vi "HAMEG_HMP2020.vi"() -> ()   [LabVIEW 2009, in "run.lvlib"]
uses:
  run.lvlib
panel:
  in  "Time":dbl[](array[numeric])
  in  "Voltage":dbl[](array[numeric])=[2.0, 2.0] format="%.3f"
  in  "Current":dbl[](array[numeric]) format="%.3f"
  in  "Channel (Channel 1)":i32(ring)=1 items=["Channel 1"=1, "Channel 2"=2, "Channel 3"=3, "Channel 4"=4]
  in  "VISA resource name":refnum<visa-resource-name>="GPIB::20::INSTR"
  in  "stop":bool
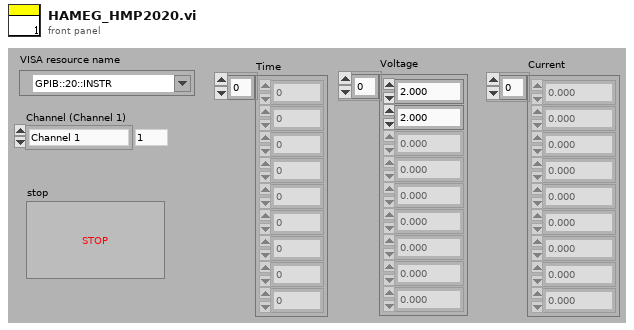
[diagram p1: front panel]
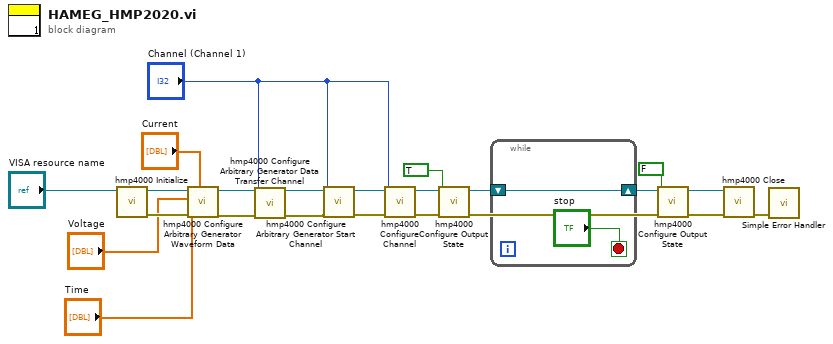
[diagram p0: block diagram]
diagram:
  n1 = call <instrlib>:"hmp4000 Initialize.vi"("VISA resource name"="VISA resource name") -> ("error out"=w22:errorcluster, "VISA resource name out"=w23:refnum<visa-resource-name>)  [unwired: 9 in]
  n2 = call <instrlib>:"hmp4000 Configure Arbitrary Generator Waveform Data.vi"("Current"="Current", "error in (no error)"=w22, "Time"="Time", "Voltage"="Voltage", "VISA resource name"=w23) -> ("error out"=w20:errorcluster, "VISA resource name out"=w21:refnum<visa-resource-name>)  [unwired: 5 in]
  n3 = call <instrlib>:"hmp4000 Configure Arbitrary Generator Data Transfer Channel.vi"("error in (no error)"=w20, "Channel (Channel 1)"="Channel (Channel 1)", "VISA resource name"=w21) -> ("error out"=w18:errorcluster, "VISA resource name out"=w19:refnum<visa-resource-name>)  [unwired: 7 in]
  n4 = call <instrlib>:"hmp4000 Configure Arbitrary Generator Start Channel.vi"("error in (no error)"=w18, "Channel (Channel 1)"="Channel (Channel 1)", "VISA resource name"=w19) -> ("error out"=w17:errorcluster, "VISA resource name out"=w16:refnum<visa-resource-name>)  [unwired: 7 in]
  n5 = call <instrlib>:"hmp4000 Configure Channel.vi"("error in (no error)"=w17, "Channel (Channel 1)"="Channel (Channel 1)", "VISA resource name"=w16) -> ("error out"=w15:errorcluster, "VISA resource name out"=w14:refnum<visa-resource-name>)  [unwired: 7 in]
  n6 = call <instrlib>:"hmp4000 Configure Output State.vi"("error in (no error)"=w15, "Output State (Off)"=TRUE, "VISA resource name"=w14) -> ("error out"=w13:errorcluster, "VISA resource name out"=w10:refnum<visa-resource-name>)  [unwired: 7 in]
  n7 = while {
    shift-right: [w25] -> w9
    shift-left: w10 -> [w25]
    stop <- "stop" stop-if-true
  }
  n8 = call <instrlib>:"hmp4000 Configure Output State.vi"("error in (no error)"=w13, "Output State (Off)"=FALSE, "VISA resource name"=w9) -> ("error out"=w11:errorcluster, "VISA resource name out"=w12:refnum<visa-resource-name>)  [unwired: 7 in]
  n9 = call <instrlib>:"hmp4000 Close.vi"("error in (no error)"=w11, "VISA resource name"=w12) -> ("error out"=w1:errorcluster)  [unwired: 9 in]
  n10 = call <vilib>:"Simple Error Handler.vi"("error in (no error)"=w1) -> ()  [unwired: 4 in, 5 out]
